vi "CustomerTestData.vi"() -> ()   [LabVIEW 2013]
uses:
  <vilib>/Utility/file.llb/Write To Spreadsheet File (string).vi
panel:
  in  "Array 2":bool[](array[boolean])
  out "RecordSet":string[][](array[string])
  out "query":string
  in  "work order":string
  out "Selected columns":string
  in  "Done":bool
  in  "Array":bool[](array[boolean])
  out "Column Names":string[](array[string])=["work_order", "btw_sn", "mac", "meid", "operator", "date_time", "part_number", "imei", "sim_id", "phone_number", "test_result", "board_sn", "test_time", "test_program", "test_version", "extra1", "extra2", "guid", "extra3", "extra4", "extra5", "extra6", "extra7"]
  out "Error out":errorcluster
  in  "Error in (no error)":errorcluster
  # "Include"
  # "Sort By"
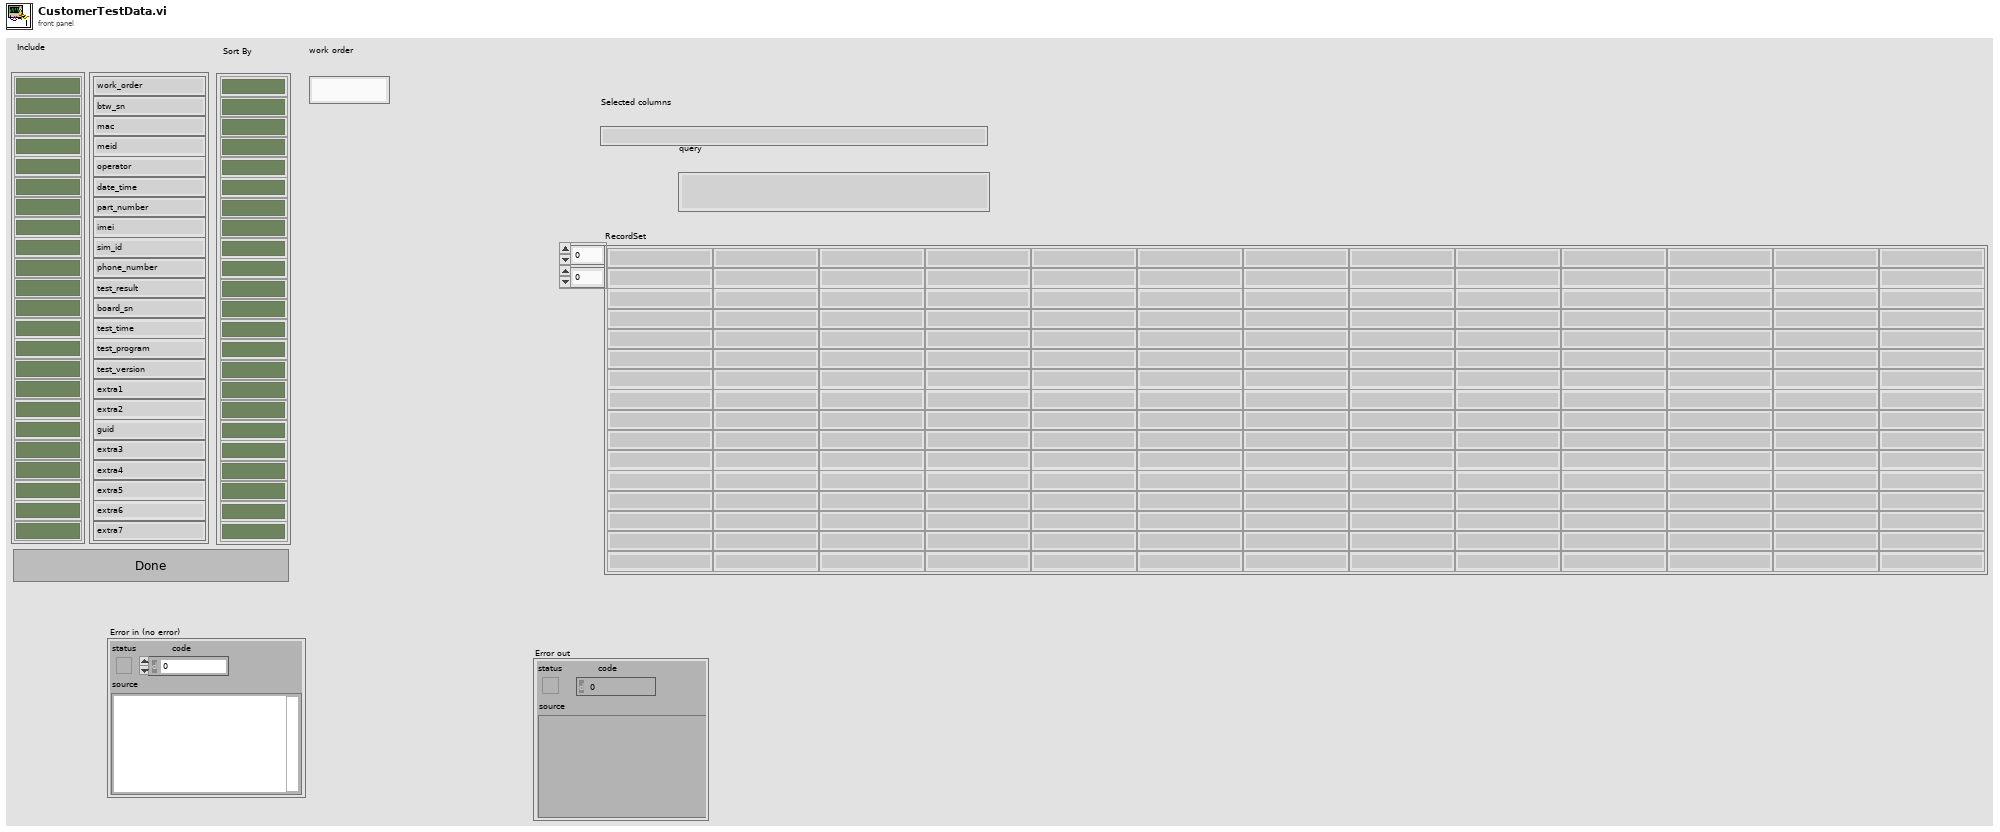
[diagram p1: front panel]
types:
  T1 = enum16{"Query", "Insert", "Select", "Dump Recs", "Get Rec Count", "Get Col Names", "Insert all fields", "Find", "Get last test result", "Get work order qty", "Set work order qty", "Save test report", "Get test report", "Execute query no data", "Select count", "Query and return row 0 col 0"}
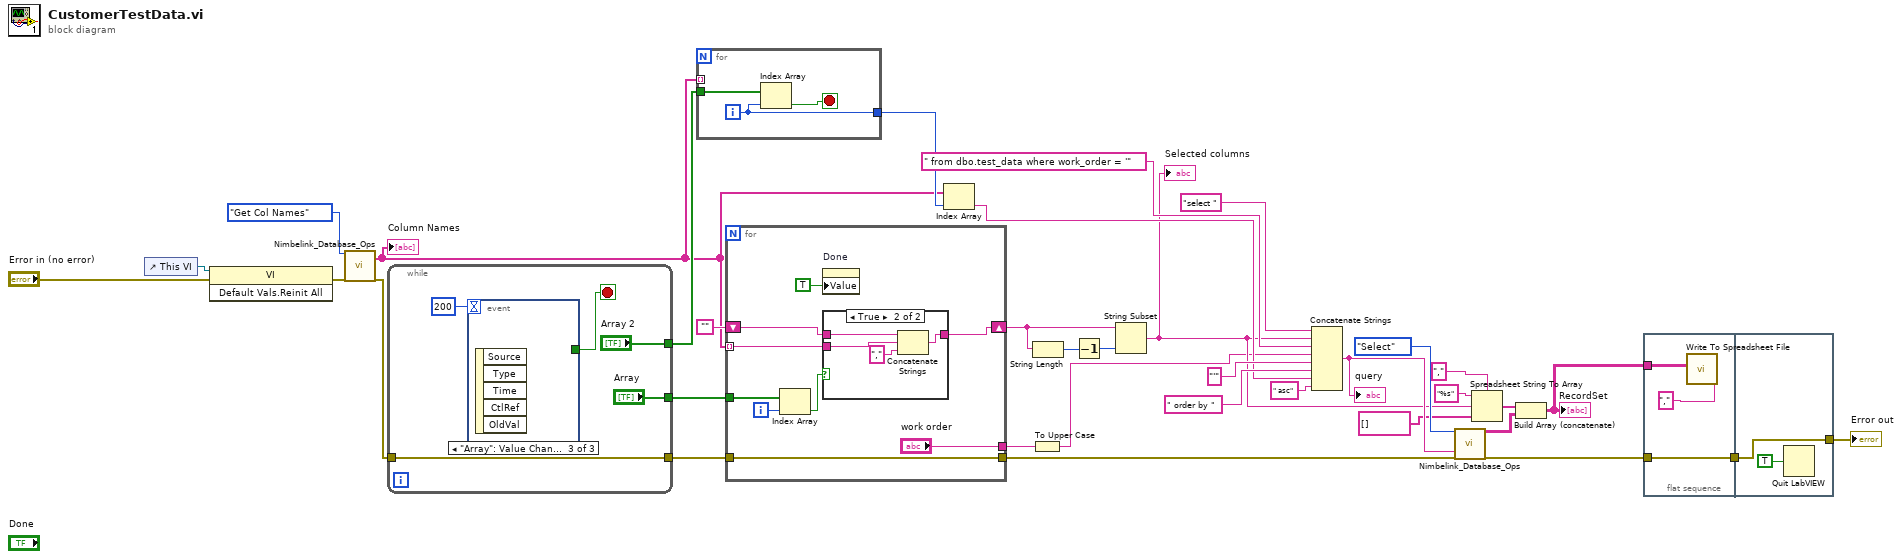
[diagram p0: block diagram]
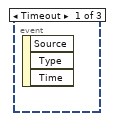
[diagram p3: hidden frame]
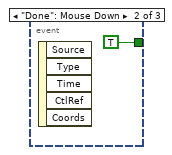
[diagram p4: hidden frame]
diagram:
  n1 = control-ref of="This VI"() -> (w30:refnum<vi>)
  n2 = invoke class="VI" method="Default Vals.Reinit All"(reference=w30, error in="Error in (no error)") -> (error out=w29:errorcluster)  [unwired: 1 in, 2 out]
  n3 = call "Nimbelink_Database_Ops.vi"("Operation"=T1."Get Col Names", "Error in (no error)"=w29) -> ("Column Names"=w13:string[], "Error out"=w34:errorcluster)  [unwired: 10 in, 6 out]
  "Column Names" <- w13
  n4 = while {
    tunnel: w34 -> [w39]
    tunnel: [w39] -> w32
    tunnel: ["Array"] -> w19
    tunnel: ["Array 2"] -> w17
    stop <- w40 stop-if-true
    n5 = event shown="[2] \"Array\": Value Change" {
      selector: _ -> [_ _ _]
      dyn-events: _ -> [_ _ _]
      timeout: 200 -> [_ _ _]
      tunnel: [_ TRUE _] -> w40
      event Timeout {
        n6 = event-data() -> ()  [unwired: 1 in, 3 out]
      }
      event "Done": Mouse Down {
        n7 = event-data() -> ()  [unwired: 1 in, 5 out]
      }
      event "Array": Value Change {
        n8 = event-data() -> ()  [unwired: 1 in, 5 out]
      }
    }
  }
  n9 = for {
    tunnel: w17 -> [w44]
    tunnel: [w42] -> w16
    tunnel: w13 -> [_] mode=indexing
    i -> [w42]
    stop <- w43 stop-if-true
    n10 = Index Array(array=w44, index=w42) -> (element=w43:bool)
  }
  n11 = for {
    tunnel: w13 -> [w49] mode=indexing
    tunnel: w19 -> [w53]
    shift-right: [w48] -> w28
    shift-left: "" -> [w50]
    tunnel: w32 -> [w47]
    tunnel: [w47] -> w20
    tunnel: ["work order"] -> w5
    i -> [w52]
    n12 = Index Array(array=w53, index=w52) -> (element=w51:bool)
    n13 = property on="Done" class="Bool (strict)"("Value"=TRUE) -> ()  [unwired: 2 in, 2 out]
    n14 = case shown="True" w51 {
      tunnel: w50 -> [w54 w58]
      tunnel: w49 -> [_ w57]
      tunnel: [w54 w55] -> w48
      frame False {
      }
      frame True {
        n15 = Concatenate Strings(w58, w57, "," ("string")) -> (w55:string)
      }
    }
  }
  n16 = Index Array(array=w13, index=w16) -> (element=w15:string)
  n17 = To Upper Case(1:w5) -> (0:w4:string)
  n18 = String Length(string=w28) -> (length=w27:i32)
  n19 = Decrement(x=w27) -> (x-1=w26:i32)
  n20 = String Subset(string=w28, length (rest)=w26) -> (substring=w12:string)  [unwired: 1 in]
  "Selected columns" <- w12
  n21 = Concatenate Strings("select " ("string"), w12, " from dbo.test_data where work_order = '" ("string"), w4, "'" ("string"), " order by " ("string"), w15, " asc" ("string")) -> (w21:string)
  "query" <- w21
  n22 = call "Nimbelink_Database_Ops.vi"("Operation"=T1."Select", "SQL Query"=w21, "Error in (no error)"=w20) -> ("RecordSet"=w7:string[][], "Error out"=w3:errorcluster)  [unwired: 9 in, 6 out]
  n23 = Spreadsheet String To Array(delimiter (Tab)=",", format string="%s", spreadsheet string=w12, array type (2D Dbl)=string[] []) -> (array=w8:string[])
  n24 = Build Array (concatenate)(w8, w7) -> (w6:string[][])
  "RecordSet" <- w6
  n25 = flat-sequence {
    tunnel: w6 -> [w60]
    tunnel: w3 -> [w59]
    tunnel: [w59] -> w2
    tunnel: [w62] -> w1
    tunnel: w2 -> [w62]
    frame #0 {
      n26 = call-poly <vilib>:"Write To Spreadsheet File.vi"("delimiter (\\t)"="," ("delimiter (\\t)"), "2D data"=w60) -> ()  [unwired: 6 in, 1 out]
    }
    frame #1 {
      n27 = Quit LabVIEW(quit? (T)=TRUE) -> ()
    }
  }
  "Error out" <- w1
